vi "Periodic Tasks.vi"() -> ()   [LabVIEW 2014]
doc: "This VI runs in parallel to other tasks. It can contain as many user-defined periodic loops as you need. These can carry out PID or other sorts of timed response."
uses:
  <vilib>/Rock Robotics/WPI/DriverStation/WPI_DriverStationRobotMode2.ctl
  NavX Code/navX-MXP Library/COMMON/TypeDefs/Value TypeDefs/navX Device Registers.ctl
  Global Variables.vi
  Robot Global Data.vi
  <vilib>/addons/control/pid/pid.llb/PID (DBL).vi
  <vilib>/addons/control/pid/NI_PID_pid.lvlib
  <vilib>/Rock Robotics/WPI/DriverStation/WPI_DriverStationStatusErrorCache.ctl
  NavX Code/navX-MXP Library/navX-MXP IMU.lvlib
  <vilib>/Utility/file.llb/Write To Spreadsheet File (DBL).vi
  <vilib>/Utility/file.llb/Read From Spreadsheet File (DBL).vi
panel:
  out "Heading":cluster{"X":dbl, "Y":dbl}[](graph)
  out "Yaw":cluster{"X":dbl, "Y":dbl}[](graph)
  out "Roll":cluster{"X":dbl, "Y":dbl}[](graph)
  out "Pitch":cluster{"X":dbl, "Y":dbl}[](graph)
  in  "Angle":dbl=5.0 format="%#_13g"
  out "Robot Y":dbl
  out "Robot X":dbl
  in  "On Ramp":bool
  in  "Stationary Gryo":dbl
  in  "PID gains":T1={"proportional gain (Kc)"=0.02, "integral time (Ti, min)"=0.0, "derivative time (Td, min)"=0.0} {"derivative time (Td, min)" format="%.3f"; "integral time (Ti, min)" format="%.3f"; "proportional gain (Kc)" format="%.3f"}
  out "Valid?":bool
  out "Offset":dbl
  in  "Left Rumble":sgl
  in  "Right Rumble":sgl
  out "navX Data":u8[](array[numeric])
  in  "PID gains":T1={"proportional gain (Kc)"=1.0, "integral time (Ti, min)"=0.01, "derivative time (Td, min)"=0.0} {"derivative time (Td, min)" format="%.3f"; "integral time (Ti, min)" format="%.3f"; "proportional gain (Kc)" format="%.3f"}
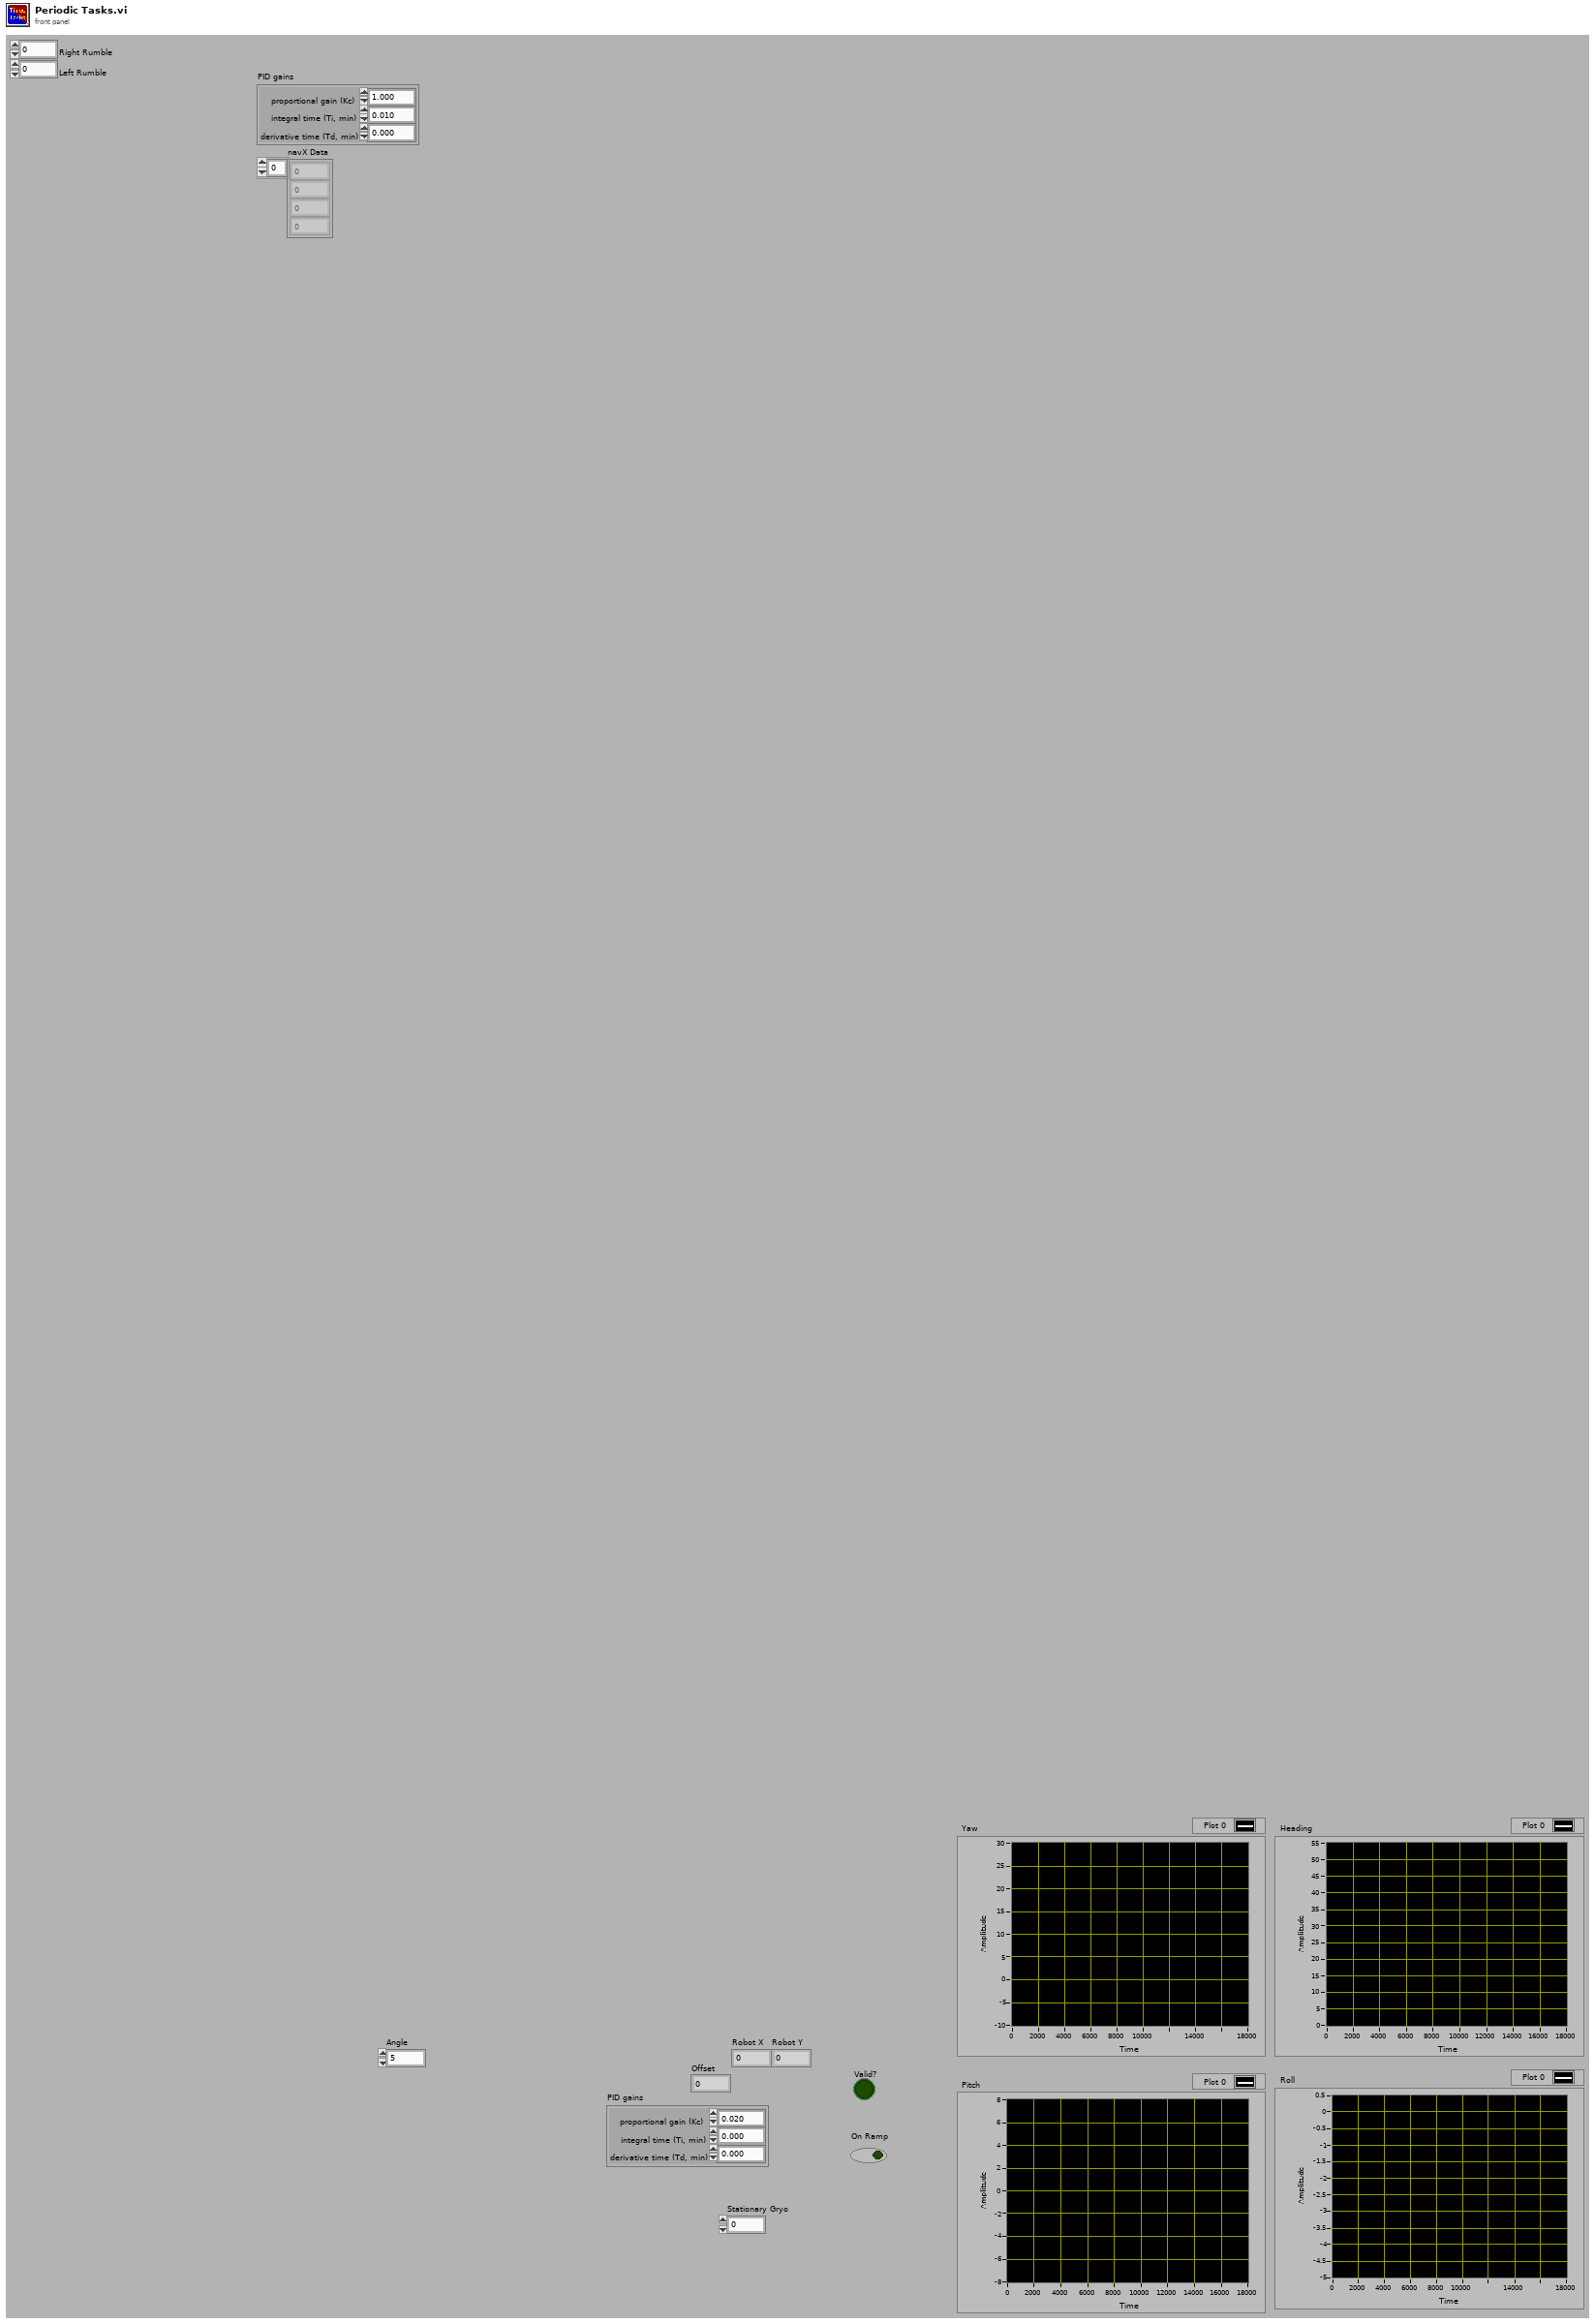
[diagram p1: front panel]
types:
  T1 = cluster{"proportional gain (Kc)":dbl, "integral time (Ti, min)":dbl, "derivative time (Td, min)":dbl}
  T2 = enum16{"Stop", "Three Tote", "Two Tote", "One Tote", "Step", "Top", "Home", "Joystick"}
  T3 = typedef "WPI_JoystickDevRef.ctl" = cluster{"Device":T4}
  T4 = typedef "WPI_JoystickDeviceEnum.ctl" = enum16{"USB 0", "USB 1", "USB 2", "USB 3", "USB 4", "USB 5"}
  T5 = typedef "navX-MXP IMU.lvlib/navX Device Registers.ctl" = u8
  T6 = typedef "navX-MXP IMU.lvlib/navX Device TypeDef.ctl" = cluster{"navX Interface Protocol":T7, "navX Interface Protocol TypeDefs":cluster{"SPIDevRef":T8, "I2CDevRef":T11}, "navX System Information":cluster{"Board Information":T13, "Status":T14, "Offsets":T18}, "navX Common Information":cluster{"Update Rate (4Hz-60Hz)":T19, "refnum name":string, "error":errorcluster}}
  T7 = typedef "navX-MXP IMU.lvlib/navX Interface Protocol.ctl" = enum16{"SPI", "I2C"}
  T8 = typedef "WPI_SPIDevRef.ctl" = cluster{"DevStatus":errorcluster, "Handle":i32, "Controller":T9, "SPI Bus":T10}
  T9 = typedef "FPGA_TypedefDigitalModule.ctl" = enum16{"Controller 1"}
  T10 = typedef "spi_bus.ctl" = enum16{"SPI On-Board, CS0", "SPI On-Board, CS1", "SPI On-Board, CS2", "SPI On-Board, CS3", "SPI MXP", "Invalid"}
  T11 = typedef "WPI_I2CDevRef.ctl" = cluster{"DevStatus":errorcluster, "Controller":T9, "Device Address":u8, "Handle":i32, "I2C Bus":T12}
  T12 = typedef "i2c_bus.ctl" = enum16{"I2C On-Board", "I2C MXP", "Invalid"}
  T13 = typedef "navX-MXP IMU.lvlib/navX Board Information.ctl" = cluster{"WhoAmI (50 | 0x32)":u8, "Board Revision":u8, "Firmware Major Version":u8, "Firmware Minor Version":u8}
  T14 = typedef "navX-MXP IMU.lvlib/navX Status Data.ctl" = cluster{"Update Rate Hz":u8, "Accelerometer Full-Scale Range":u8, "Gyro Full-Scale Range":u16, "NAVX_OP_STATUS":T15, "NAVX_CAL_STATUS":T16, "NAVX_SELFTEST_STATUS":u8, "NAVX_SENSOR_STATUS":T17}
  T15 = typedef "navX-MXP IMU.lvlib/navX NAVX_OP_STATUS.ctl" = u8
  T16 = typedef "navX-MXP IMU.lvlib/navX NAVX_CAL_STATUS.ctl" = u8
  T17 = typedef "navX-MXP IMU.lvlib/navX NAVX_SENSOR_STATUS.ctl" = cluster{"MOVING":bool, "YAW_STABLE":bool, "MAG_DISTURBANCE":bool, "ALTITUDE_VALID":bool, "SEALEVEL_PRESS_SET":bool, "FUSED_HEADING_VALID":bool}
  T18 = typedef "navX-MXP IMU.lvlib/navX Offsets Data.ctl" = cluster{"Yaw":dbl, "Quat W":dbl, "Quat X":dbl, "Quat Y":dbl, "Quat Z":dbl}
  T19 = typedef "navX-MXP IMU.lvlib/navX Update Rate.ctl" = u8
  T20 = typedef "WPI_DriverStationStatusErrorCache.ctl" = enum16{"Get", "Set"}
  T21 = typedef "WPI_MotorControlDeviceRef.ctl" = cluster{"DeviceStatus":errorcluster, "Type":T22, "PWM":cluster{"Controller":T9, "PWM Channel":T23, "DeadBand":T24}, "CAN":cluster{"Device Number":u8, "Control Mode":T25, "Semaphore":T26, "Max Vout":dbl, "TalonSRX Control Mode":T27}, "Invert":bool, "TransformRef":T28, "InvTransformRef":T28}
  T22 = typedef "WPI_MotorControlType.ctl" = enum16{"PWM", "CAN", "CANTalonSRX"}
  T23 = typedef "FPGA_DIOPWMChannel.ctl" = enum8{"PWM 0", "PWM 1", "PWM 2", "PWM 3", "PWM 4", "PWM 5", "PWM 6", "PWM 7", "PWM 8", "PWM 9", "PWM MXP 0", "PWM MXP 1", "PWM MXP 2", "PWM MXP 3", "PWM MXP 4", "PWM MXP 5", "PWM MXP 6", "PWM MXP 7", "PWM MXP 8", "PWM MXP 9", "Invalid"}
  T24 = typedef "WPI_PWMDeadband.ctl" = cluster{"Name":string, "maxPositivePwm":i32, "minPositivePwm":i32, "centerPwm":i32, "maxNegativePwm":i32, "minNegativePwm":i32, "angularRange":u16}
  T25 = typedef "WPI_CANJaguar_ControlMode.ctl" = enum8{"Percent VBus", "Current", "Speed", "Position", "Voltage"}
  T26 = typedef "Semaphore RefNum" = refnum<k1>
  T27 = typedef "WPI_CANTalonSRX_APIControlMode.ctl" = enum8{"Percent VBus", "Speed", "Position", "Slave", "Unchanged / Invalid"}
  T28 = typedef "WPI_PWMTransform_ConPane.ctl" = refnum<vi>
  T29 = typedef "WPI_DriverStationRobotMode2.ctl" = enum16{"Autonomous Disabled", "Autonomous Enabled", "Teleop Disabled", "Teleop Enabled", "Disconnected", "Finish", "Test Disabled", "Test Enabled", "Emergency Stopped"}
  T30 = typedef "navX-MXP IMU.lvlib/navX Vector Data.ctl" = cluster{"X":dbl, "Y":dbl, "Z":dbl}
  T31 = typedef "navX-MXP IMU.lvlib/navX YPRH Data.ctl" = cluster{"Yaw":dbl, "Pitch":dbl, "Roll":dbl, "Heading":dbl}
  T32 = typedef "WPI_CounterDevRef.ctl" = cluster{"DevStatus":errorcluster, "CntIndex":T33}
  T33 = typedef "FPGA_CounterCtrSystemIndex.ctl" = enum8{"Ctr 0", "Ctr 1", "Ctr 2", "Ctr 3", "Ctr 4", "Ctr 5", "Ctr 6", "Ctr 7", "Invalid"}
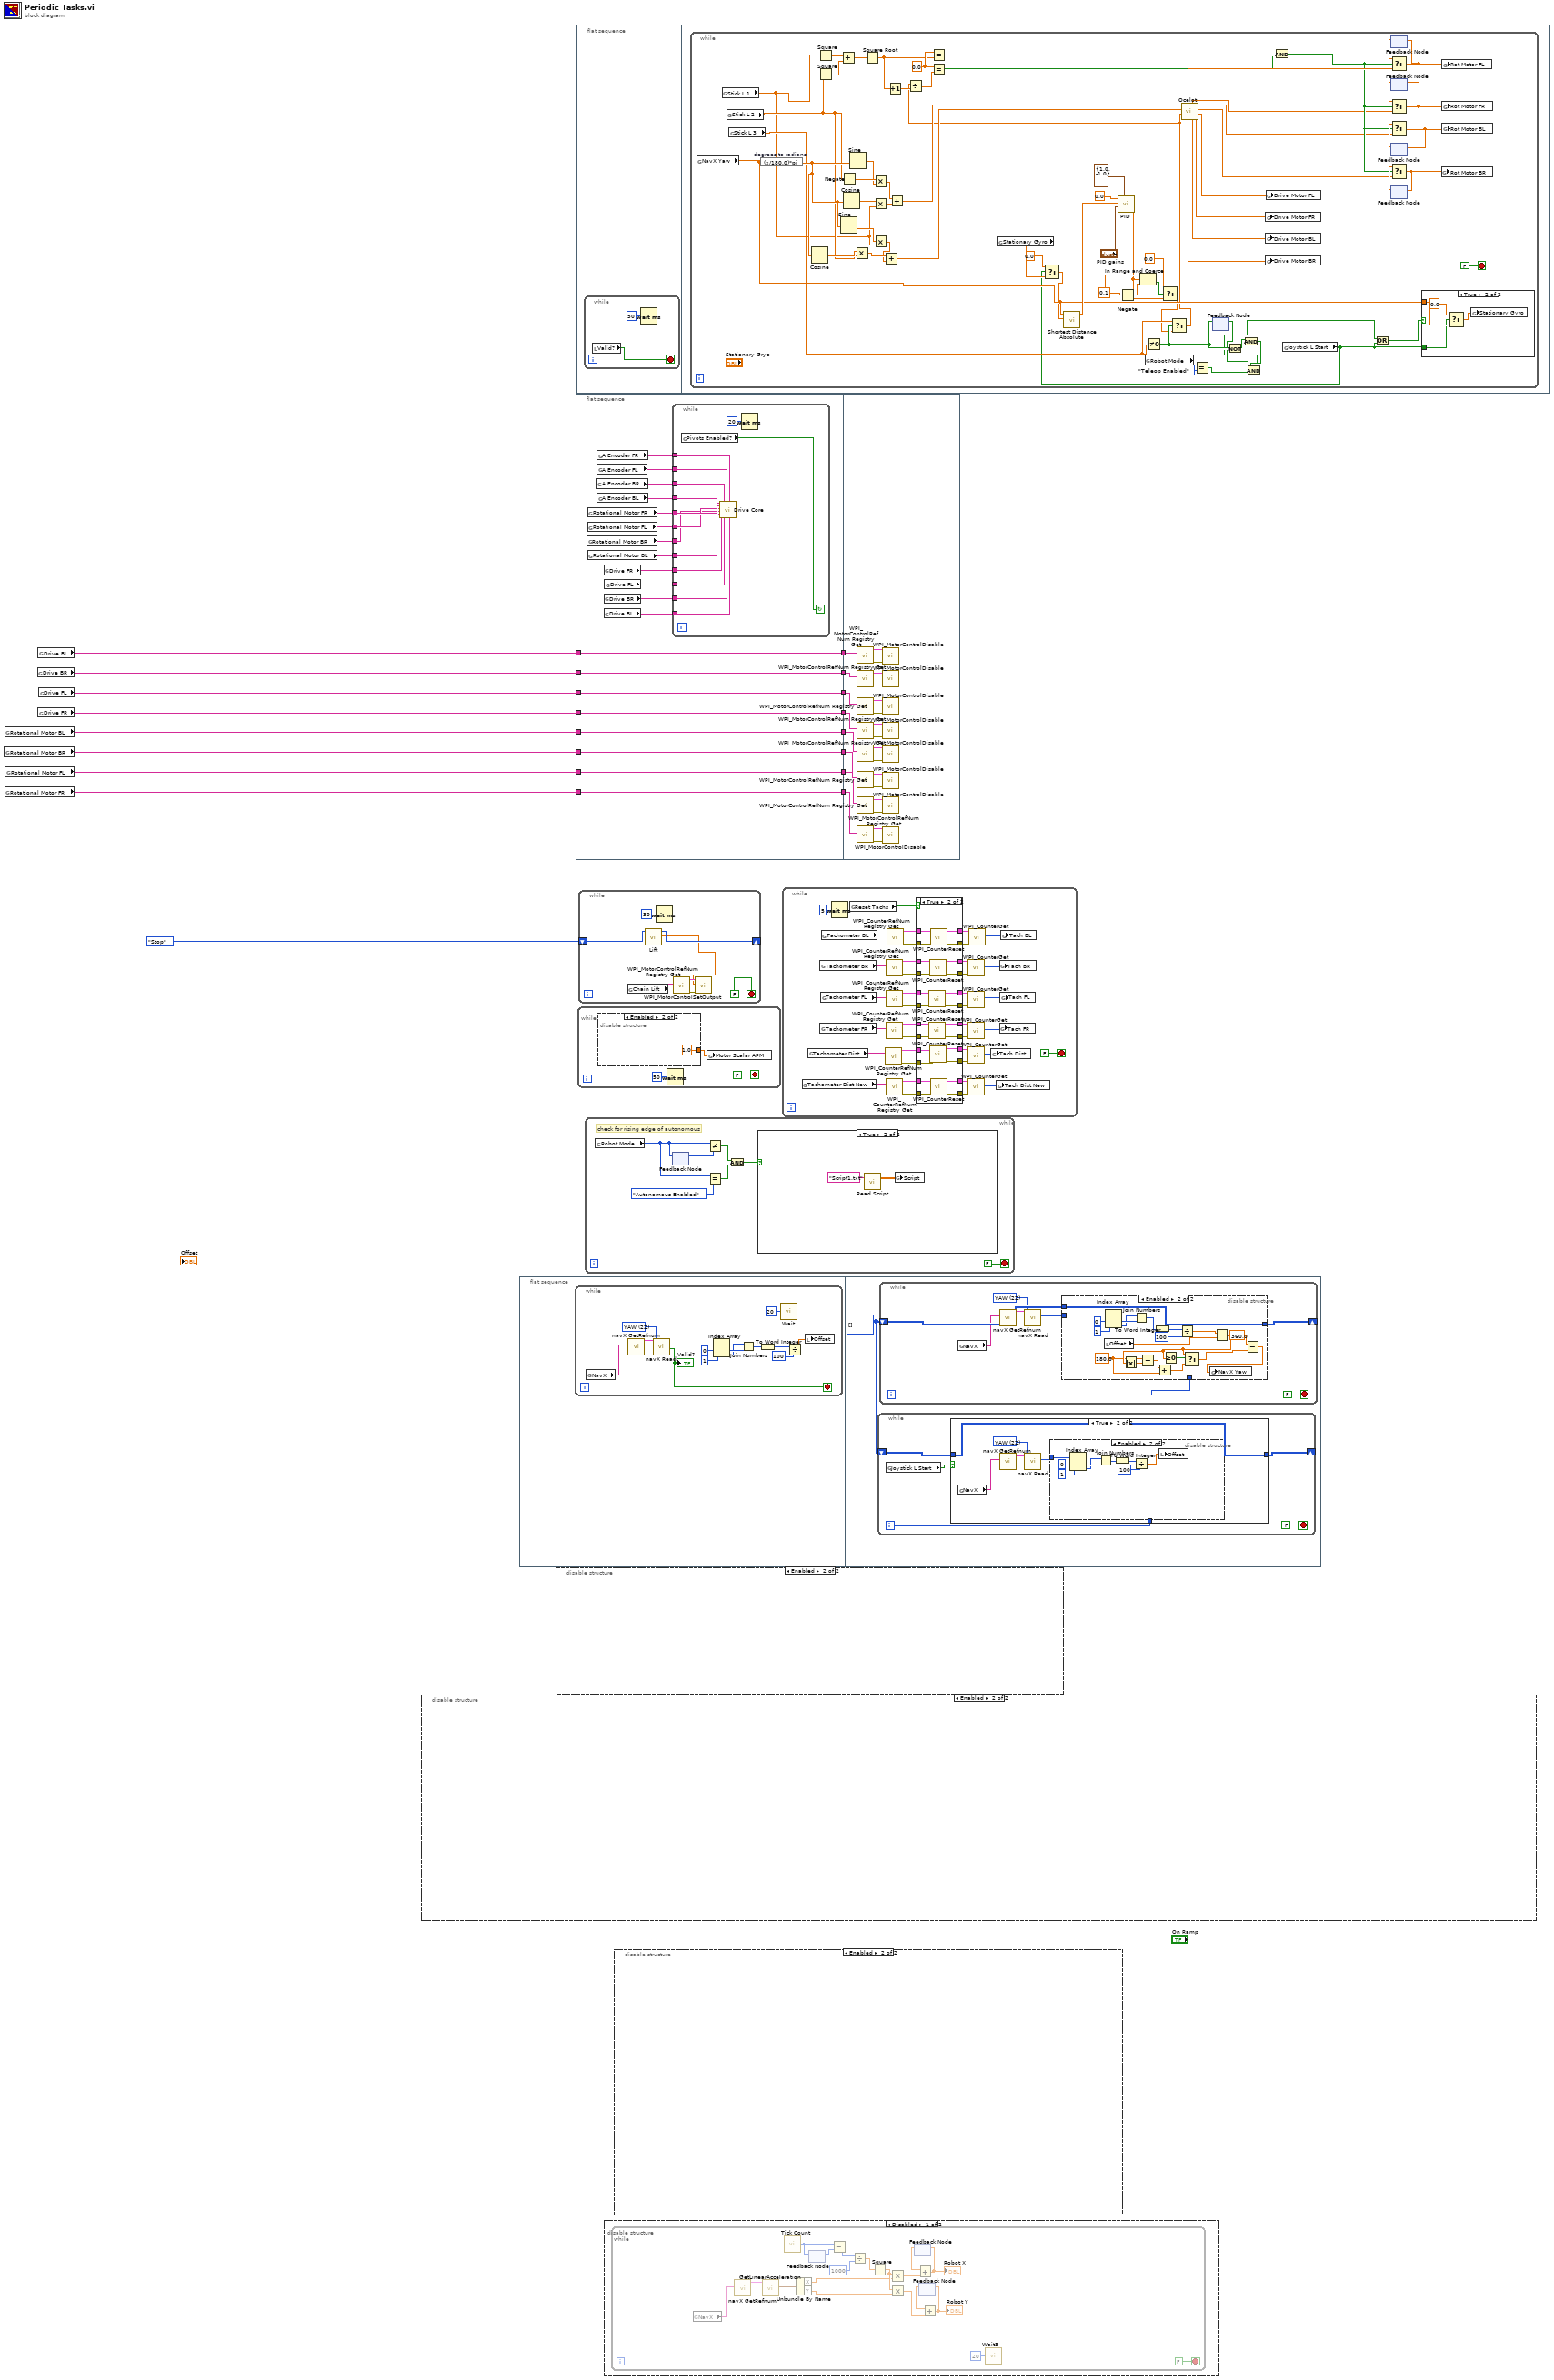
[diagram p0: block diagram]
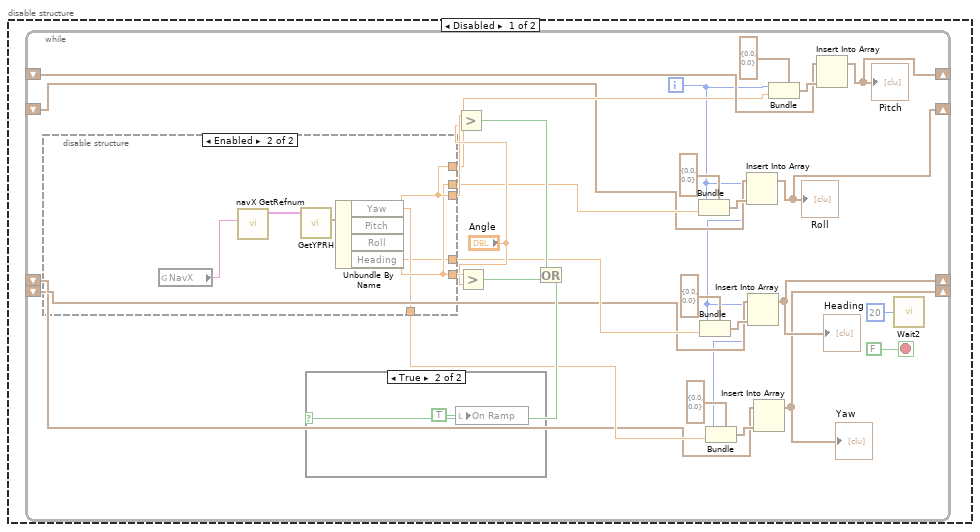
[diagram p4: hidden frame]
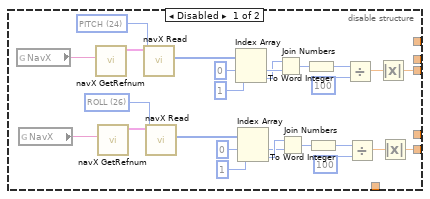
[diagram p5: hidden frame]
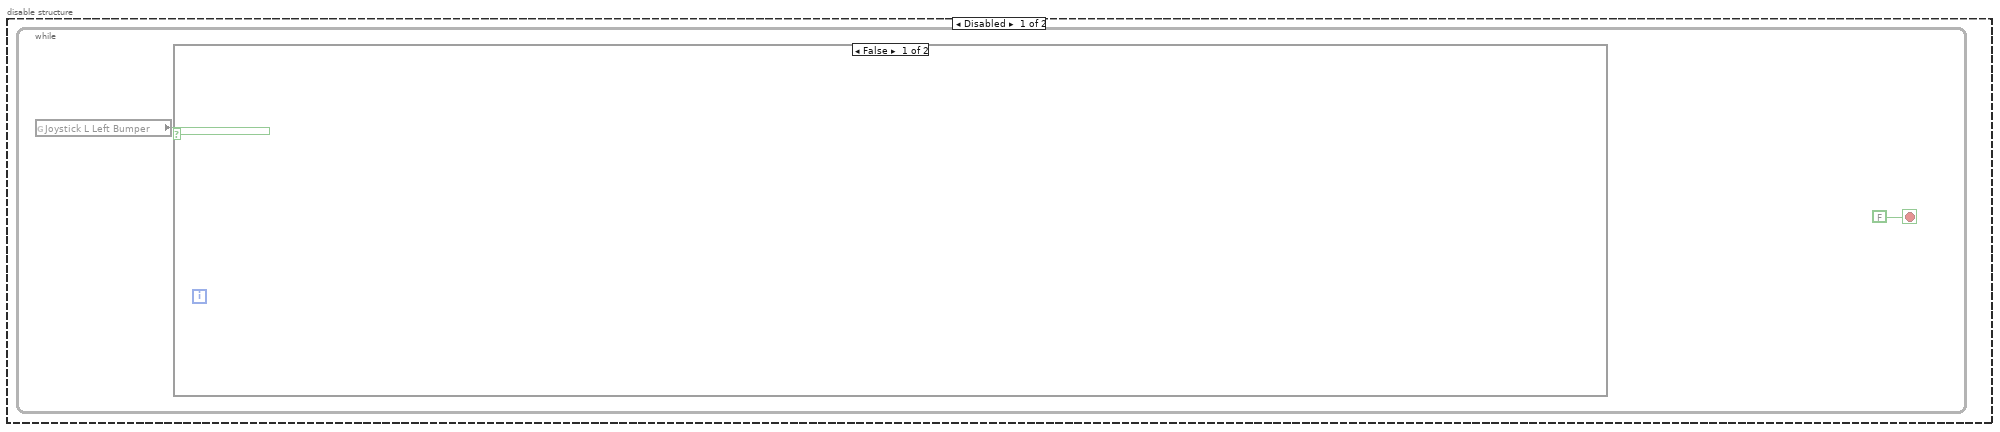
[diagram p7: hidden frame]
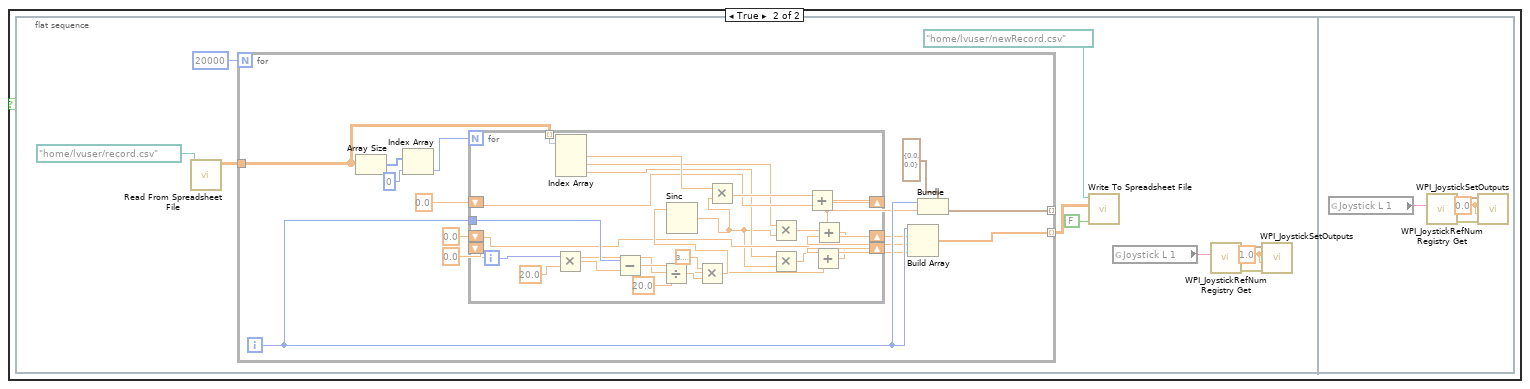
[diagram p8: hidden frame]
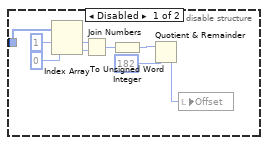
[diagram p10: hidden frame]
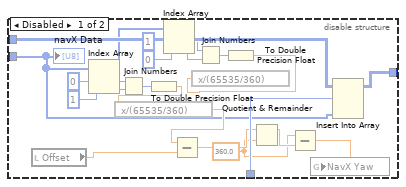
[diagram p11: hidden frame]
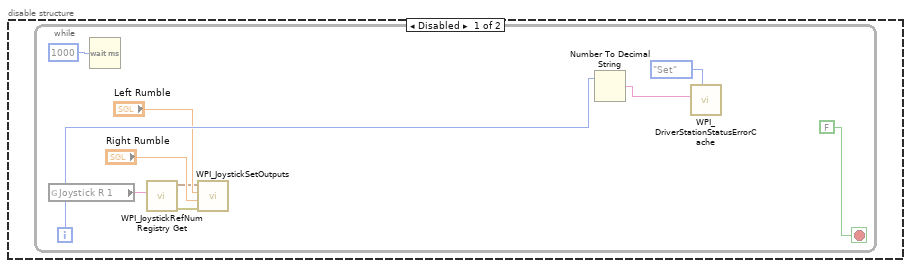
[diagram p12: hidden frame]
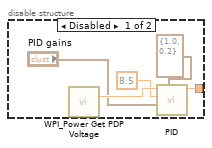
[diagram p15: hidden frame]
diagram:
  n1 = global read "Global Variables.vi" "Rotational Motor BR"() -> (w6:string)
  n2 = global read "Global Variables.vi" "Rotational Motor BL"() -> (w8:string)
  n3 = global read "Global Variables.vi" "Rotational Motor FR"() -> (w2:string)
  n4 = global read "Global Variables.vi" "Rotational Motor FL"() -> (w4:string)
  n5 = global read "Global Variables.vi" "Drive BR"() -> (w14:string)
  n6 = global read "Global Variables.vi" "Drive BL"() -> (w16:string)
  n7 = global read "Global Variables.vi" "Drive FR"() -> (w10:string)
  n8 = global read "Global Variables.vi" "Drive FL"() -> (w12:string)
  n9 = disable-structure shown="Enabled" {
    frame Disabled {
      n10 = while {
        stop <- FALSE stop-if-true
        n11 = global read "Global Variables.vi" "Joystick L Left Bumper"() -> (w18:bool)
        n12 = case shown="False" w18 {
          frame False {
          }
          frame True {
            n13 = flat-sequence {
              frame #0 {
                w23 = sgl 1.0 ("Left Rumble")
                n14 = call-poly <vilib>:"Read From Spreadsheet File.vi"("file path (dialog if empty)"=path "/home/lvuser/record.csv") -> ("all rows"=w28:dbl[][])  [unwired: 6 in, 4 out]
                n15 = for {
                  N: 20000 -> [_]
                  tunnel: [w38] -> _ mode=indexing
                  tunnel: w28 -> [w37]
                  tunnel: [w34] -> w27 mode=indexing
                  i -> [w36]
                  n16 = Array Size(array=w37) -> (size(s)=w43:i32[])
                  n17 = Index Array(array=w43, index=0) -> (element=w42:i32)
                  n18 = for {
                    N: w42 -> [_]
                    shift-right: [w53] -> w35
                    shift-left: 0.0 -> [w55]
                    tunnel: w37 -> [w64] mode=indexing
                    tunnel: w36 -> [w56]
                    shift-right: [w51] -> w33
                    shift-left: 0.0 -> [w48]
                    shift-right: [w52] -> w32
                    shift-left: 0.0 -> [w47]
                    i -> [w62]
                    n19 = Multiply(x=w62, y=20.0) -> (x*y=w59:dbl)
                    n20 = Index Array(array=w64) -> (element #1=w65:dbl, element #2=w46:dbl, element #3=w45:dbl)  [unwired: 3 in]
                    n21 = Subtract(x=w56, y=w59) -> (x-y=w61:dbl)
                    n22 = Divide(x=w61, y=20.0) -> (x/y=w58:dbl)
                    n23 = Multiply(x=3.141592653589793, y=w58) -> (x*y=w54:dbl)
                    n24 = Sinc(1:w54) -> (0:w44:dbl)
                    n25 = Multiply(x=w65, y=w44) -> (x*y=w66:dbl)
                    n26 = Multiply(x=w46, y=w44) -> (x*y=w49:dbl)
                    n27 = Multiply(x=w45, y=w44) -> (x*y=w50:dbl)
                    n28 = Add(x=w66, y=w55) -> (x+y=w53:dbl)
                    n29 = Add(x=w50, y=w47) -> (x+y=w52:dbl)
                    n30 = Add(x=w49, y=w48) -> (x+y=w51:dbl)
                  }
                  n31 = Build Array(w36, w35, w33, w32) -> (w34:dbl[])
                  n32 = Bundle(cluster=cluster{dbl, dbl} {0.0, 0.0}, w36, w35) -> (w38:cluster{dbl, dbl})
                }
                n33 = call-poly <vilib>:"Write To Spreadsheet File.vi"("append to file? (new file:F)"=FALSE, "2D data"=w27, "file path (dialog if empty)"=path "/home/lvuser/newRecord.csv") -> ()  [unwired: 5 in, 1 out]
                n34 = global read "Global Variables.vi" "Joystick L 1"() -> (w21:string)
                n35 = call <vilib>:"WPI_JoystickRefNum Registry Get.vi"("refnum name"=w21) -> ("error out"=w20:errorcluster, "JoystickDevRef"=w22:T3)  [unwired: 9 in]
                n36 = call <vilib>:"WPI_JoystickSetOutputs.vi"("error in (no error)"=w20, "Right Rumble"=w23, "Left Rumble"=w23, "JoystickDevRef"=w22) -> ()  [unwired: 6 in, 2 out]
              }
              frame #1 {
                w67 = sgl 0.0 ("Left Rumble")
                n37 = global read "Global Variables.vi" "Joystick L 1"() -> (w69:string)
                n38 = call <vilib>:"WPI_JoystickRefNum Registry Get.vi"("refnum name"=w69) -> ("error out"=w70:errorcluster, "JoystickDevRef"=w68:T3)  [unwired: 9 in]
                n39 = call <vilib>:"WPI_JoystickSetOutputs.vi"("error in (no error)"=w70, "Right Rumble"=w67, "Left Rumble"=w67, "JoystickDevRef"=w68) -> ()  [unwired: 6 in, 2 out]
              }
            }
          }
        }
      }
    }
    frame Enabled {
    }
  }
  n40 = flat-sequence {
    frame #0 {
      n41 = while {
        stop <- w72 stop-if-true
        w84 = T5 22 items=["WHOAMI"=0, "HW_REV"=1, "FW_VER_MAJOR"=2, "FW_VER_MINOR"=3, "UPDATE_RATE_HZ"=4, "ACCEL_FSR_G"=5, "GYRO_FSR_DPS"=6, "OP_STATUS"=8, "CAL_STATUS"=9, "SELFTEST_STATUS"=10, "SENSOR_STATUS"=16, "TIMESTAMP"=18, "YAW"=22, "PITCH"=24, "ROLL"=26, "HEADING"=28, "FUSED_HEADING"=30, "ALTITUDE_I"=32, "ALTITUDE_D"=34, "LINERA_ACC_X"=36, "LINERA_ACC_Y"=38, "LINERA_ACC_Z"=40, "QUAT_W"=42, "QUAT_X"=44, "QUAT_Y"=46, "QUAT_Z"=48, "MPU_TEMP_C"=50, "GYRO_X"=52, "GYRO_Y"=54, "GYRO_Z"=56, "ACC_X"=58, "ACC_Y"=60, "ACC_Z"=62, "MAG_X"=64, "MAG_Y"=66, "MAG_Z"=68, "PRESSURE_I"=70, "PRESSURE_D"=72, "PRESSURE_TEMP"=74, "YAW_OFFSET"=76, "QUAT_OFFSET_W"=78, "QUAT_OFFSET_X"=80, "QUAT_OFFSET_Y"=82, "QUAT_OFFSET_Z"=84] ("Device Register (WHOAMI)")
        n42 = global read "Global Variables.vi" "NavX"() -> (w83:string)
        n43 = call "navX GetRefnum.vi"("refnum name"=w83) -> ("navX Device TypeDef"=w82:T6)  [unwired: 9 in, 1 out]
        n44 = call "navX Read.vi"("Device Register (WHOAMI)"=w84, "navX Device TypeDef"=w82) -> ("Valid?"=w72:bool, "navX Data"=w81:u8[])  [unwired: 7 in, 1 out]
        "Valid?" <- w72
        n45 = Index Array(array=w81, index #1=0 ("index"), index #2=1 ("index")) -> (element #1=w75:u8, element #2=w74:u8)
        n46 = Join Numbers(hi=w74, lo=w75) -> ((hi.lo)=w78:u16)
        n47 = To Word Integer(number=w78) -> (16bit integer=w77:i16)
        n48 = call "Wait"("Count(mSec)"=u32 20) -> ()  [unwired: 1 out]
        n49 = Divide(x=w77, y=i16 100) -> (x/y=w71:dbl)
        n50 = local write "Offset"(w71) -> ()
      }
    }
    frame #1 {
      w85 = u16[][] []
      n51 = while {
        shift-right: [w88] -> _
        shift-left: w85 -> [w87]
        i -> [w89]
        stop <- FALSE stop-if-true
        n52 = global read "Global Variables.vi" "Joystick L Start"() -> (w86:bool)
        n53 = case shown="True" w86 {
          tunnel: w89 -> [_ _]
          tunnel: [w91 w92] -> w88
          tunnel: w87 -> [w91 w92]
          frame False {
          }
          frame True {
            w94 = T5 22 items=["WHOAMI"=0, "HW_REV"=1, "FW_VER_MAJOR"=2, "FW_VER_MINOR"=3, "UPDATE_RATE_HZ"=4, "ACCEL_FSR_G"=5, "GYRO_FSR_DPS"=6, "OP_STATUS"=8, "CAL_STATUS"=9, "SELFTEST_STATUS"=10, "SENSOR_STATUS"=16, "TIMESTAMP"=18, "YAW"=22, "PITCH"=24, "ROLL"=26, "HEADING"=28, "FUSED_HEADING"=30, "ALTITUDE_I"=32, "ALTITUDE_D"=34, "LINERA_ACC_X"=36, "LINERA_ACC_Y"=38, "LINERA_ACC_Z"=40, "QUAT_W"=42, "QUAT_X"=44, "QUAT_Y"=46, "QUAT_Z"=48, "MPU_TEMP_C"=50, "GYRO_X"=52, "GYRO_Y"=54, "GYRO_Z"=56, "ACC_X"=58, "ACC_Y"=60, "ACC_Z"=62, "MAG_X"=64, "MAG_Y"=66, "MAG_Z"=68, "PRESSURE_I"=70, "PRESSURE_D"=72, "PRESSURE_TEMP"=74, "YAW_OFFSET"=76, "QUAT_OFFSET_W"=78, "QUAT_OFFSET_X"=80, "QUAT_OFFSET_Y"=82, "QUAT_OFFSET_Z"=84] ("Device Register (WHOAMI)")
            n54 = global read "Global Variables.vi" "NavX"() -> (w95:string)
            n55 = call "navX GetRefnum.vi"("refnum name"=w95) -> ("navX Device TypeDef"=w96:T6)  [unwired: 9 in, 1 out]
            n56 = call "navX Read.vi"("Device Register (WHOAMI)"=w94, "navX Device TypeDef"=w96) -> ("navX Data"=w93:u8[])  [unwired: 7 in, 2 out]
            n57 = disable-structure shown="Enabled" {
              disable-tunnel: w93 -> [w100 w109]
              frame Disabled {
                n58 = Index Array(array=w100, index #1=1 ("index"), index #2=0 ("index")) -> (element #1=w99:u8, element #2=w98:u8)
                n59 = Join Numbers(hi=w99, lo=w98) -> ((hi.lo)=w103:u16)
                n60 = To Unsigned Word Integer(number=w103) -> (unsigned 16bit integer=w102:u16)
                n61 = Quotient & Remainder(x=w102, y=u16 182) -> (floor(x/y)=w97:u16)  [unwired: 1 out]
                n62 = local write "Offset"(w97) -> ()
              }
              frame Enabled {
                n63 = Index Array(array=w109, index #1=0 ("index"), index #2=1 ("index")) -> (element #1=w108:u8, element #2=w107:u8)
                n64 = Join Numbers(hi=w107, lo=w108) -> ((hi.lo)=w112:u16)
                n65 = To Word Integer(number=w112) -> (16bit integer=w111:i16)
                n66 = Divide(x=w111, y=i16 100) -> (x/y=w106:dbl)
                n67 = local write "Offset"(w106) -> ()
              }
            }
          }
        }
      }
      n68 = while {
        shift-right: [w120] -> _
        shift-left: w85 -> [w119]
        i -> [w121]
        stop <- FALSE stop-if-true
        w116 = T5 22 items=["WHOAMI"=0, "HW_REV"=1, "FW_VER_MAJOR"=2, "FW_VER_MINOR"=3, "UPDATE_RATE_HZ"=4, "ACCEL_FSR_G"=5, "GYRO_FSR_DPS"=6, "OP_STATUS"=8, "CAL_STATUS"=9, "SELFTEST_STATUS"=10, "SENSOR_STATUS"=16, "TIMESTAMP"=18, "YAW"=22, "PITCH"=24, "ROLL"=26, "HEADING"=28, "FUSED_HEADING"=30, "ALTITUDE_I"=32, "ALTITUDE_D"=34, "LINERA_ACC_X"=36, "LINERA_ACC_Y"=38, "LINERA_ACC_Z"=40, "QUAT_W"=42, "QUAT_X"=44, "QUAT_Y"=46, "QUAT_Z"=48, "MPU_TEMP_C"=50, "GYRO_X"=52, "GYRO_Y"=54, "GYRO_Z"=56, "ACC_X"=58, "ACC_Y"=60, "ACC_Z"=62, "MAG_X"=64, "MAG_Y"=66, "MAG_Z"=68, "PRESSURE_I"=70, "PRESSURE_D"=72, "PRESSURE_TEMP"=74, "YAW_OFFSET"=76, "QUAT_OFFSET_W"=78, "QUAT_OFFSET_X"=80, "QUAT_OFFSET_Y"=82, "QUAT_OFFSET_Z"=84] ("Device Register (WHOAMI)")
        n69 = global read "Global Variables.vi" "NavX"() -> (w117:string)
        n70 = call "navX GetRefnum.vi"("refnum name"=w117) -> ("navX Device TypeDef"=w118:T6)  [unwired: 9 in, 1 out]
        n71 = call "navX Read.vi"("Device Register (WHOAMI)"=w116, "navX Device TypeDef"=w118) -> ("navX Data"=w115:u8[])  [unwired: 7 in, 2 out]
        n72 = disable-structure shown="Enabled" {
          disable-tunnel: w121 -> [w139 _]
          disable-tunnel: [w138 w163] -> w120
          disable-tunnel: w119 -> [w137 w163]
          disable-tunnel: w115 -> [w127 w164]
          frame Disabled {
            w133 = 360.0 ("y")
            n73 = local read "Offset"() -> (w136:dbl)
            n74 = Index Array(array=w127, index #1=0 ("index"), index #2=1 ("index")) -> (element #1=w144:u8, element #2=w143:u8)
            n75 = Join Numbers(hi=w144, lo=w143) -> ((hi.lo)=w140:u16)
            n76 = To Double Precision Float(number=w140) -> (double precision float=w131:dbl)
            n77 = expression code="x/(65535/360)"(w131) -> (w130:dbl)
            n78 = Index Array(array=w127, index #1=1 ("index"), index #2=0 ("index")) -> (element #1=w125:u8, element #2=w124:u8)
            n79 = Subtract(x=w130, y=w136) -> (x-y=w135:dbl)
            n80 = Join Numbers(hi=w125, lo=w124) -> ((hi.lo)=w126:u16)
            n81 = To Double Precision Float(number=w126) -> (double precision float=w123:dbl)
            n82 = expression code="x/(65535/360)"(w123) -> ()  [unwired: 1 out]
            n83 = Quotient & Remainder(x=w135, y=w133) -> (x-y*floor(x/y)=w134:dbl)  [unwired: 1 out]
            n84 = Subtract(x=w133, y=w134) -> (x-y=w132:dbl)
            n85 = global write "Global Variables.vi" "NavX Yaw"(w132) -> ()
            n86 = Insert Into Array(array=w137, index (row)=w139, new element=w127) -> (w138:u16[][])  [unwired: 1 in]
            "navX Data" <- w127
          }
          frame Enabled {
            w148 = 180.0 ("x")
            n87 = local read "Offset"() -> (w156:dbl)
            n88 = Index Array(array=w164, index #1=0 ("index"), index #2=1 ("index")) -> (element #1=w160:u8, element #2=w159:u8)
            n89 = Join Numbers(hi=w159, lo=w160) -> ((hi.lo)=w158:u16)
            n90 = To Word Integer(number=w158) -> (16bit integer=w155:i16)
            n91 = Divide(x=w155, y=i16 100) -> (x/y=w157:dbl)
            n92 = Subtract(x=w157, y=w156) -> (x-y=w152:dbl)
            n93 = Absolute Value(x=w152) -> (abs(x)=w151:dbl)
            n94 = Subtract(x=w148, y=w151) -> (x-y=w149:dbl)
            n95 = Add(x=w149, y=w148) -> (x+y=w150:dbl)
            n96 = Greater Or Equal To 0?(x=w152) -> (x >= 0?=w153:bool)
            n97 = Select(t=w152, s=w153, f=w150) -> (s? t:f=w146:dbl)
            n98 = Subtract(x=360.0, y=w146) -> (x-y=w145:dbl)
            n99 = global write "Global Variables.vi" "NavX Yaw"(w145) -> ()
          }
        }
      }
    }
  }
  n100 = disable-structure shown="Enabled" {
    frame Disabled {
      n101 = while {
        i -> [w171]
        stop <- FALSE stop-if-true
        n102 = global read "Global Variables.vi" "Joystick R 1"() -> (w166:string)
        n103 = Wait (ms)(milliseconds to wait=u32 1000) -> ()  [unwired: 1 out]
        n104 = call <vilib>:"WPI_JoystickRefNum Registry Get.vi"("refnum name"=w166) -> ("error out"=w165:errorcluster, "JoystickDevRef"=w167:T3)  [unwired: 9 in]
        n105 = call <vilib>:"WPI_JoystickSetOutputs.vi"("error in (no error)"=w165, "Right Rumble"="Right Rumble", "Left Rumble"="Left Rumble", "JoystickDevRef"=w167) -> ()  [unwired: 6 in, 2 out]
        n106 = Number To Decimal String(number=w171) -> (decimal integer string=w172:string)  [unwired: 1 in]
        n107 = call <vilib>:"WPI_DriverStationStatusErrorCache.vi"("StatusErrorCacheOp"=WPI_DriverStationStatusErrorCache."Set", "Error String"=w172) -> ()  [unwired: 1 in, 9 out]
      }
    }
    frame Enabled {
    }
  }
  n108 = flat-sequence {
    tunnel: [w182] -> w17
    tunnel: w16 -> [w182]
    tunnel: [w181] -> w15
    tunnel: w14 -> [w181]
    tunnel: [w180] -> w13
    tunnel: w12 -> [w180]
    tunnel: [w179] -> w11
    tunnel: w10 -> [w179]
    tunnel: [w178] -> w9
    tunnel: w8 -> [w178]
    tunnel: [w177] -> w7
    tunnel: w6 -> [w177]
    tunnel: [w176] -> w5
    tunnel: w4 -> [w176]
    tunnel: [w175] -> w3
    tunnel: w2 -> [w175]
    tunnel: w17 -> [w216]
    tunnel: w15 -> [w215]
    tunnel: w13 -> [w214]
    tunnel: w11 -> [w213]
    tunnel: w9 -> [w212]
    tunnel: w7 -> [w211]
    tunnel: w5 -> [w210]
    tunnel: w3 -> [w209]
    frame #0 {
      n109 = global read "Global Variables.vi" "Rotational Motor BR"() -> (w188:string)
      n110 = global read "Global Variables.vi" "Rotational Motor FR"() -> (w190:string)
      n111 = global read "Global Variables.vi" "Rotational Motor FL"() -> (w189:string)
      n112 = global read "Global Variables.vi" "Rotational Motor BL"() -> (w187:string)
      n113 = global read "Global Variables.vi" "A Encoder BR"() -> (w192:string)
      n114 = global read "Global Variables.vi" "A Encoder FR"() -> (w194:string)
      n115 = global read "Global Variables.vi" "A Encoder FL"() -> (w193:string)
      n116 = global read "Global Variables.vi" "A Encoder BL"() -> (w191:string)
      n117 = global read "Global Variables.vi" "Drive FR"() -> (w186:string)
      n118 = global read "Global Variables.vi" "Drive BR"() -> (w184:string)
      n119 = global read "Global Variables.vi" "Drive BL"() -> (w183:string)
      n120 = global read "Global Variables.vi" "Drive FL"() -> (w185:string)
      n121 = while {
        tunnel: w194 -> [w207]
        tunnel: w193 -> [w206]
        tunnel: w192 -> [w205]
        tunnel: w191 -> [w204]
        tunnel: w190 -> [w203]
        tunnel: w189 -> [w202]
        tunnel: w188 -> [w201]
        tunnel: w187 -> [w200]
        tunnel: w186 -> [w199]
        tunnel: w185 -> [w198]
        tunnel: w184 -> [w197]
        tunnel: w183 -> [w196]
        stop <- w208 continue-if-true
        n122 = global read "Global Variables.vi" "Pivots Enabled?"() -> (w208:bool)
        n123 = call "Drive Core.vi"("A Encoder BL"=w204, "Rotational Motor FR"=w203, "Rotational Motor FL"=w202, "Rotational Motor BR"=w201, "Rotational Motor BL"=w200, "Drive Motor FR"=w199, "A Encoder BR"=w205, "Drive Motor FL"=w198, "A Encoder FL"=w206, "Drive Motor BR"=w197, "A Encoder FR"=w207, "Drive Motor BL"=w196) -> ()  [unwired: 8 in]
        n124 = Wait (ms)(milliseconds to wait=u32 20) -> ()  [unwired: 1 out]
      }
    }
    frame #1 {
      n125 = call <vilib>:"WPI_MotorControlRefNum Registry Get.vi"("refnum name"=w216) -> ("error out"=w232:errorcluster, "MotorControlDevRef"=w231:T21)  [unwired: 9 in]
      n126 = call <vilib>:"WPI_MotorControlRefNum Registry Get.vi"("refnum name"=w215) -> ("error out"=w230:errorcluster, "MotorControlDevRef"=w229:T21)  [unwired: 9 in]
      n127 = call <vilib>:"WPI_MotorControlRefNum Registry Get.vi"("refnum name"=w214) -> ("error out"=w228:errorcluster, "MotorControlDevRef"=w227:T21)  [unwired: 9 in]
      n128 = call <vilib>:"WPI_MotorControlRefNum Registry Get.vi"("refnum name"=w213) -> ("error out"=w226:errorcluster, "MotorControlDevRef"=w225:T21)  [unwired: 9 in]
      n129 = call <vilib>:"WPI_MotorControlRefNum Registry Get.vi"("refnum name"=w212) -> ("error out"=w224:errorcluster, "MotorControlDevRef"=w223:T21)  [unwired: 9 in]
      n130 = call <vilib>:"WPI_MotorControlRefNum Registry Get.vi"("refnum name"=w211) -> ("error out"=w222:errorcluster, "MotorControlDevRef"=w221:T21)  [unwired: 9 in]
      n131 = call <vilib>:"WPI_MotorControlRefNum Registry Get.vi"("refnum name"=w210) -> ("error out"=w220:errorcluster, "MotorControlDevRef"=w219:T21)  [unwired: 9 in]
      n132 = call <vilib>:"WPI_MotorControlRefNum Registry Get.vi"("refnum name"=w209) -> ("error out"=w218:errorcluster, "MotorControlDevRef"=w217:T21)  [unwired: 9 in]
      n133 = call <vilib>:"WPI_MotorControlDisable.vi"("error in (no error)"=w232, "MotorControlDevRef"=w231) -> ()  [unwired: 8 in, 2 out]
      n134 = call <vilib>:"WPI_MotorControlDisable.vi"("error in (no error)"=w230, "MotorControlDevRef"=w229) -> ()  [unwired: 8 in, 2 out]
      n135 = call <vilib>:"WPI_MotorControlDisable.vi"("error in (no error)"=w228, "MotorControlDevRef"=w227) -> ()  [unwired: 8 in, 2 out]
      n136 = call <vilib>:"WPI_MotorControlDisable.vi"("error in (no error)"=w226, "MotorControlDevRef"=w225) -> ()  [unwired: 8 in, 2 out]
      n137 = call <vilib>:"WPI_MotorControlDisable.vi"("error in (no error)"=w224, "MotorControlDevRef"=w223) -> ()  [unwired: 8 in, 2 out]
      n138 = call <vilib>:"WPI_MotorControlDisable.vi"("error in (no error)"=w222, "MotorControlDevRef"=w221) -> ()  [unwired: 8 in, 2 out]
      n139 = call <vilib>:"WPI_MotorControlDisable.vi"("error in (no error)"=w220, "MotorControlDevRef"=w219) -> ()  [unwired: 8 in, 2 out]
      n140 = call <vilib>:"WPI_MotorControlDisable.vi"("error in (no error)"=w218, "MotorControlDevRef"=w217) -> ()  [unwired: 8 in, 2 out]
    }
  }
  n141 = flat-sequence {
    frame #0 {
      n142 = while {
        stop <- w234 stop-if-true
        n143 = local read "Valid?"() -> (w234:bool)
        n144 = Wait (ms)(milliseconds to wait=u32 50) -> ()  [unwired: 1 out]
      }
    }
    frame #1 {
      n145 = while {
        stop <- FALSE stop-if-true
        w246 = 0.1 ("Value to Deadband (default of 0.1)")
        w298 = 0.0 ("x")
        n146 = global read "Global Variables.vi" "NavX Yaw"() -> (w253:dbl)
        n147 = global read "Global Variables.vi" "Stick L 1"() -> (w235:dbl)
        n148 = global read "Global Variables.vi" "Stick L 2"() -> (w259:dbl)
        n149 = global read "Global Variables.vi" "Stick L 3"() -> (w258:dbl)
        n150 = expression code="(x/180.0)*pi" "degrees to radians"(w253) -> (w267:dbl)
        n151 = Cosine(x=w267) -> (cos(x)=w266:dbl)
        n152 = Square(x=w235) -> (x^2=w300:dbl)
        n153 = Square(x=w259) -> (x^2=w301:dbl)
        n154 = Add(x=w300, y=w301) -> (x+y=w299:dbl)
        n155 = Sine(x=w267) -> (sin(x)=w274:dbl)
        n156 = Negate(x=w259) -> (-x=w273:dbl)
        n157 = Cosine(x=w267) -> (cos(x)=w271:dbl)
        n158 = Sine(x=w267) -> (sin(x)=w268:dbl)
        n159 = Multiply(x=w266, y=w259) -> (x*y=w265:dbl)
        n160 = Square Root(x=w299) -> (sqrt(x)=w297:dbl)
        n161 = Multiply(x=w273, y=w268) -> (x*y=w272:dbl)
        n162 = Multiply(x=w271, y=w235) -> (x*y=w270:dbl)
        n163 = Multiply(x=w274, y=w235) -> (x*y=w264:dbl)
        n164 = Add(x=w265, y=w264) -> (x+y=w263:dbl)
        n165 = Increment(x=w297) -> (x+1=w296:dbl)
        n166 = Add(x=w272, y=w270) -> (x+y=w269:dbl)
        n167 = Equal?(x=w298, y=w297) -> (x = y?=w289:bool)
        n168 = global read "Global Variables.vi" "Stationary Gyro"() -> (w237:dbl)
        n169 = Negate(x=w246) -> (-x=w247:dbl)
        n170 = global read "Robot Global Data.vi" "Robot Mode"() -> (w251:T29)
        n171 = Not Equal To 0?(x=w258) -> (x != 0?=w255:bool)
        n172 = Equal?(x=w251, y=WPI_DriverStationRobotMode2."Teleop Enabled") -> (x = y?=w249:bool)
        n173 = feedback #1() -> (w254:bool)  [unwired: 1 in]
        n174 = feedback-in #1(w255) -> ()
        n175 = Not(x=w255) -> (.not. x?=w256:bool)
        n176 = And(x=w256, y=w254) -> (x .and. y?=w248:bool)
        n177 = And(x=w248, y=w249) -> (x .and. y?=w241:bool)
        n178 = global read "Global Variables.vi" "Joystick L Start"() -> (w236:bool)
        n179 = Select(t=0.0, s=w236, f=w237) -> (s? t:f=w238:dbl)
        n180 = call "Shortest Distance Absolute.vi"("Target"=w238, "Current"=w253) -> ("Angle to Rotate"=w257:dbl)  [unwired: 9 in]
        n181 = call-poly <vilib>:"PID.vi"("output range"=cluster{"output high":dbl, "output low":dbl} {"output high"=1.0, "output low"=-1.0}, "PID gains"="PID gains", "process variable"=w257, "setpoint"=0.0) -> ("output"=w243:dbl)  [unwired: 6 in, 1 out]
        n182 = In Range and Coerce(upper limit=w246, x=w243, lower limit=w247) -> (In Range?=w245:bool)  [unwired: 1 out]
        n183 = Select(t=0.0, s=w245, f=w243) -> (s? t:f=w242:dbl)
        n184 = Select(t=w258, s=w255, f=w242) -> (s? t:f=w252:dbl)
        n185 = Divide(x=w252, y=w296) -> (x/y=w295:dbl)
        n186 = Equal?(x=w298, y=w295) -> (x = y?=w288:bool)
        n187 = call "Ocelot.vi"("RCW (X2)"=w252, "FWD (Y)"=w263, "STR (X)"=w269) -> ("FRD"=w278:dbl, "FLD"=w279:dbl, "BRS"=w280:dbl, "BLS"=w281:dbl, "BLD"=w277:dbl, "FRS"=w282:dbl, "BRD"=w276:dbl, "FLS"=w290:dbl)  [unwired: 1 in]
        n188 = global write "Global Variables.vi" "Drive Motor FR"(w278) -> ()
        n189 = global write "Global Variables.vi" "Drive Motor BL"(w277) -> ()
        n190 = global write "Global Variables.vi" "Drive Motor BR"(w276) -> ()
        n191 = global write "Global Variables.vi" "Drive Motor FL"(w279) -> ()
        n192 = And(x=w289, y=w288) -> (x .and. y?=w287:bool)
        n193 = Or(x=w241, y=w236) -> (x .or. y?=w240:bool)
        n194 = feedback #2() -> (w294:dbl)  [unwired: 1 in]
        n195 = Select(t=w294, s=w287, f=w290) -> (s? t:f=w286:dbl)
        n196 = feedback-in #2(w286) -> ()
        n197 = feedback #3() -> (w293:dbl)  [unwired: 1 in]
        n198 = Select(t=w293, s=w287, f=w282) -> (s? t:f=w285:dbl)
        n199 = feedback-in #3(w285) -> ()
        n200 = feedback #4() -> (w292:dbl)  [unwired: 1 in]
        n201 = Select(t=w292, s=w287, f=w281) -> (s? t:f=w284:dbl)
        n202 = feedback-in #4(w284) -> ()
        n203 = feedback #5() -> (w291:dbl)  [unwired: 1 in]
        n204 = Select(t=w291, s=w287, f=w280) -> (s? t:f=w283:dbl)
        n205 = feedback-in #5(w283) -> ()
        n206 = case shown="True" w240 {
          tunnel: w253 -> [_ w305]
          tunnel: w236 -> [_ w304]
          frame False {
          }
          frame True {
            n207 = Select(t=0.0, s=w304, f=w305) -> (s? t:f=w302:dbl)
            n208 = global write "Global Variables.vi" "Stationary Gyro"(w302) -> ()
          }
        }
        n209 = global write "Global Variables.vi" "Rot Motor BR"(w283) -> ()
        n210 = global write "Global Variables.vi" "Rot Motor FL"(w286) -> ()
        n211 = global write "Global Variables.vi" "Rot Motor FR"(w285) -> ()
        n212 = global write "Global Variables.vi" "Rot Motor BL"(w284) -> ()
      }
    }
  }
  n213 = while {
    stop <- FALSE stop-if-true
    n214 = disable-structure shown="Enabled" {
      disable-tunnel: [w309 1.0 ("Motor Scalar APM")] -> w306
      frame Disabled {
        n215 = call <vilib>:"WPI_Power Get PDP Voltage.vi"() -> ("voltage (V)"=w312:dbl)  [unwired: 14 in, 1 out]
        n216 = call-poly <vilib>:"PID.vi"("output range"=cluster{"output high":dbl, "output low":dbl} {"output high"=1.0, "output low"=0.2}, "PID gains"="PID gains", "process variable"=8.5 ("setpoint"), "setpoint"=w312) -> ("output"=w309:dbl)  [unwired: 6 in, 1 out]
      }
      frame Enabled {
      }
    }
    n217 = Wait (ms)(milliseconds to wait=u32 50) -> ()  [unwired: 1 out]
    n218 = global write "Global Variables.vi" "Motor Scalar APM"(w306) -> ()
  }
  n219 = while {
    shift-right: [w320] -> _
    shift-left: T2."Stop" ("State Out") -> [w321]
    stop <- FALSE stop-if-true
    n220 = global read "Global Variables.vi" "Chain Lift"() -> (w315:string)
    n221 = call "Lift.vi"("State"=w321) -> ("Lift Motor(Global...)"=w316:dbl, "State Out"=w320:T2)  [unwired: 9 in]
    n222 = Wait (ms)(milliseconds to wait=u32 30) -> ()  [unwired: 1 out]
    n223 = call <vilib>:"WPI_MotorControlRefNum Registry Get.vi"("refnum name"=w315) -> ("error out"=w319:errorcluster, "MotorControlDevRef"=w318:T21)  [unwired: 9 in]
    n224 = call <vilib>:"WPI_MotorControlSetOutput.vi"("error in (no error)"=w319, "Output"=w316, "MotorControlDevRef"=w318) -> ()  [unwired: 6 in, 3 out]
  }
  n225 = while {
    stop <- FALSE stop-if-true
    # "check for rising edge of autonomous"
    n226 = global read "Robot Global Data.vi" "Robot Mode"() -> (w327:T29)
    n227 = feedback #6() -> (w329:T29)  [unwired: 1 in]
    n228 = feedback-in #6(w327) -> ()
    n229 = Not Equal?(x=w327, y=w329) -> (x != y?=w325:bool)
    n230 = Equal?(x=w327, y=WPI_DriverStationRobotMode2."Autonomous Enabled" ("Robot Mode")) -> (x = y?=w326:bool)
    n231 = And(x=w325, y=w326) -> (x .and. y?=w323:bool)
    n232 = case shown="True" w323 {
      frame False {
      }
      frame True {
        n233 = call "Read Script.vi"("script name"="Script1.txt") -> ("output array"=w330:dbl[][])  [unwired: 1 in, 1 out]
        n234 = global write "Global Variables.vi" "Script"(w330) -> ()
      }
    }
  }
  n235 = disable-structure shown="Disabled" {
    frame Disabled {
      n236 = while {
        stop <- FALSE stop-if-true
        n237 = global read "Global Variables.vi" "NavX"() -> (w349:string)
        n238 = call "navX GetRefnum.vi"("refnum name"=w349) -> ("navX Device TypeDef"=w348:T6)  [unwired: 9 in, 1 out]
        n239 = call "GetLinearAcceleration.vi"("navX Device TypeDef"=w348) -> ("Linear Acceleration"=w347:T30)  [unwired: 8 in, 2 out]
        n240 = call "Tick Count"() -> ("Tick Count(mSec)"=w343:u32)
        n241 = Unbundle By Name(w347) -> ("X"=w340:dbl, "Y"=w339:dbl)
        n242 = feedback-in #7(w343) -> ()
        n243 = feedback #7() -> (w342:u32)  [unwired: 1 in]
        n244 = Subtract(x=w343, y=w342) -> (x-y=w344:u32)
        n245 = Divide(x=w344, y=u32 1000) -> (x/y=w346:dbl)
        n246 = Square(x=w346) -> (x^2=w341:dbl)
        n247 = Multiply(x=w341, y=w340) -> (x*y=w338:dbl)
        n248 = Multiply(x=w341, y=w339) -> (x*y=w334:dbl)
        n249 = feedback #8() -> (w336:dbl)  [unwired: 1 in]
        n250 = Add(x=w336, y=w338) -> (x+y=w337:dbl)
        "Robot X" <- w337
        n251 = feedback-in #8(w337) -> ()
        n252 = feedback #9() -> (w335:dbl)  [unwired: 1 in]
        n253 = Add(x=w335, y=w334) -> (x+y=w333:dbl)
        "Robot Y" <- w333
        n254 = feedback-in #9(w333) -> ()
        n255 = call "Wait3"("Count(mSec)"=u32 20) -> ()  [unwired: 1 out]
      }
    }
    frame Enabled {
    }
  }
  n256 = disable-structure shown="Enabled" {
    frame Disabled {
      n257 = while {
        shift-right: [w369] -> _
        shift-left: _ -> [w368]
        shift-right: [w363] -> _
        shift-left: _ -> [w362]
        shift-right: [w352] -> _
        shift-left: _ -> [w355]
        shift-right: [w351] -> _
        shift-left: _ -> [w354]
        i -> [w353]
        stop <- FALSE stop-if-true
        n258 = disable-structure shown="Enabled" {
          disable-tunnel: [w394 w409] -> w378
          disable-tunnel: [w391 w408] -> w374
          disable-tunnel: [_ w409] -> w367
          disable-tunnel: [_ w408] -> w364
          disable-tunnel: [_ w407] -> w357
          disable-tunnel: [_ w406] -> w356
          frame Disabled {
            w382 = T5 26 items=["WHOAMI"=0, "HW_REV"=1, "FW_VER_MAJOR"=2, "FW_VER_MINOR"=3, "UPDATE_RATE_HZ"=4, "ACCEL_FSR_G"=5, "GYRO_FSR_DPS"=6, "OP_STATUS"=8, "CAL_STATUS"=9, "SELFTEST_STATUS"=10, "SENSOR_STATUS"=16, "TIMESTAMP"=18, "YAW"=22, "PITCH"=24, "ROLL"=26, "HEADING"=28, "FUSED_HEADING"=30, "ALTITUDE_I"=32, "ALTITUDE_D"=34, "LINERA_ACC_X"=36, "LINERA_ACC_Y"=38, "LINERA_ACC_Z"=40, "QUAT_W"=42, "QUAT_X"=44, "QUAT_Y"=46, "QUAT_Z"=48, "MPU_TEMP_C"=50, "GYRO_X"=52, "GYRO_Y"=54, "GYRO_Z"=56, "ACC_X"=58, "ACC_Y"=60, "ACC_Z"=62, "MAG_X"=64, "MAG_Y"=66, "MAG_Z"=68, "PRESSURE_I"=70, "PRESSURE_D"=72, "PRESSURE_TEMP"=74, "YAW_OFFSET"=76, "QUAT_OFFSET_W"=78, "QUAT_OFFSET_X"=80, "QUAT_OFFSET_Y"=82, "QUAT_OFFSET_Z"=84] ("Device Register (WHOAMI)")
            w403 = T5 24 items=["WHOAMI"=0, "HW_REV"=1, "FW_VER_MAJOR"=2, "FW_VER_MINOR"=3, "UPDATE_RATE_HZ"=4, "ACCEL_FSR_G"=5, "GYRO_FSR_DPS"=6, "OP_STATUS"=8, "CAL_STATUS"=9, "SELFTEST_STATUS"=10, "SENSOR_STATUS"=16, "TIMESTAMP"=18, "YAW"=22, "PITCH"=24, "ROLL"=26, "HEADING"=28, "FUSED_HEADING"=30, "ALTITUDE_I"=32, "ALTITUDE_D"=34, "LINERA_ACC_X"=36, "LINERA_ACC_Y"=38, "LINERA_ACC_Z"=40, "QUAT_W"=42, "QUAT_X"=44, "QUAT_Y"=46, "QUAT_Z"=48, "MPU_TEMP_C"=50, "GYRO_X"=52, "GYRO_Y"=54, "GYRO_Z"=56, "ACC_X"=58, "ACC_Y"=60, "ACC_Z"=62, "MAG_X"=64, "MAG_Y"=66, "MAG_Z"=68, "PRESSURE_I"=70, "PRESSURE_D"=72, "PRESSURE_TEMP"=74, "YAW_OFFSET"=76, "QUAT_OFFSET_W"=78, "QUAT_OFFSET_X"=80, "QUAT_OFFSET_Y"=82, "QUAT_OFFSET_Z"=84] ("Device Register (WHOAMI)")
            n259 = global read "Global Variables.vi" "NavX"() -> (w404:string)
            n260 = global read "Global Variables.vi" "NavX"() -> (w381:string)
            n261 = call "navX GetRefnum.vi"("refnum name"=w404) -> ("navX Device TypeDef"=w405:T6)  [unwired: 9 in, 1 out]
            n262 = call "navX GetRefnum.vi"("refnum name"=w381) -> ("navX Device TypeDef"=w380:T6)  [unwired: 9 in, 1 out]
            n263 = call "navX Read.vi"("Device Register (WHOAMI)"=w403, "navX Device TypeDef"=w405) -> ("navX Data"=w395:u8[])  [unwired: 7 in, 2 out]
            n264 = call "navX Read.vi"("Device Register (WHOAMI)"=w382, "navX Device TypeDef"=w380) -> ("navX Data"=w390:u8[])  [unwired: 7 in, 2 out]
            n265 = Index Array(array=w395, index #1=0 ("index"), index #2=1 ("index")) -> (element #1=w397:u8, element #2=w396:u8)
            n266 = Index Array(array=w390, index #1=0 ("index"), index #2=1 ("index")) -> (element #1=w388:u8, element #2=w389:u8)
            n267 = Join Numbers(hi=w396, lo=w397) -> ((hi.lo)=w400:u16)
            n268 = Join Numbers(hi=w389, lo=w388) -> ((hi.lo)=w385:u16)
            n269 = To Word Integer(number=w400) -> (16bit integer=w399:i16)
            n270 = To Word Integer(number=w385) -> (16bit integer=w386:i16)
            n271 = Divide(x=w399, y=i16 100) -> (x/y=w393:dbl)
            n272 = Divide(x=w386, y=i16 100) -> (x/y=w392:dbl)
            n273 = Absolute Value(x=w393) -> (abs(x)=w394:dbl)
            n274 = Absolute Value(x=w392) -> (abs(x)=w391:dbl)
          }
          frame Enabled {
            n275 = global read "Global Variables.vi" "NavX"() -> (w411:string)
            n276 = call "navX GetRefnum.vi"("refnum name"=w411) -> ("navX Device TypeDef"=w410:T6)  [unwired: 9 in, 1 out]
            n277 = call "GetYPRH.vi"("navX Device TypeDef"=w410) -> ("YPRH"=w412:T31)  [unwired: 8 in, 2 out]
            n278 = Unbundle By Name(w412) -> ("Yaw"=w407:dbl, "Pitch"=w409:dbl, "Roll"=w408:dbl, "Heading"=w406:dbl)
          }
        }
        n279 = Greater?(x=w378, y="Angle") -> (0:w376:bool)
        n280 = Greater?(x=w374, y="Angle") -> (0:w373:bool)
        n281 = Or(x=w376, y=w373) -> (x .or. y?=w375:bool)
        n282 = case shown="True" w375 {
          frame False {
          }
          frame True {
            n283 = local write "On Ramp"(TRUE ("On Ramp")) -> ()
          }
        }
        n284 = Bundle(cluster=cluster{"Pitch":dbl, "Roll":dbl} {"Pitch"=0.0, "Roll"=0.0}, "Pitch"=w353, "Roll"=w364) -> (w365:cluster{"Pitch":dbl, "Roll":dbl})
        n285 = Bundle(cluster=cluster{"Pitch":dbl, "Roll":dbl} {"Pitch"=0.0, "Roll"=0.0}, "Pitch"=w353, "Roll"=w356) -> (w361:cluster{"Pitch":dbl, "Roll":dbl})
        n286 = Bundle(cluster=cluster{"Pitch":dbl, "Roll":dbl} {"Pitch"=0.0, "Roll"=0.0}, "Pitch"=w353, "Roll"=w357) -> (w358:cluster{"Pitch":dbl, "Roll":dbl})
        n287 = Insert Into Array(array=w362, new element=w365) -> (w363:cluster{"Pitch":dbl, "Roll":dbl}[])  [unwired: 1 in]
        "Roll" <- w363
        n288 = Insert Into Array(array=w355, new element=w361) -> (w352:cluster{"Pitch":dbl, "Roll":dbl}[])  [unwired: 1 in]
        "Heading" <- w352
        n289 = Insert Into Array(array=w354, new element=w358) -> (w351:cluster{"Pitch":dbl, "Roll":dbl}[])  [unwired: 1 in]
        "Yaw" <- w351
        n290 = Bundle(cluster=cluster{"Pitch":dbl, "Roll":dbl} {"Pitch"=0.0, "Roll"=0.0}, "Pitch"=w353, "Roll"=w367) -> (w370:cluster{"Pitch":dbl, "Roll":dbl})
        n291 = Insert Into Array(array=w368, new element=w370) -> (w369:cluster{"Pitch":dbl, "Roll":dbl}[])  [unwired: 1 in]
        "Pitch" <- w369
        n292 = call "Wait2"("Count(mSec)"=u32 20) -> ()  [unwired: 1 out]
      }
    }
    frame Enabled {
    }
  }
  n293 = while {
    stop <- FALSE stop-if-true
    n294 = global read "Global Variables.vi" "Tachometer Dist New"() -> (w420:string)
    n295 = global read "Global Variables.vi" "Tachometer Dist"() -> (w424:string)
    n296 = global read "Global Variables.vi" "Tachometer BR"() -> (w440:string)
    n297 = global read "Global Variables.vi" "Tachometer FR"() -> (w428:string)
    n298 = global read "Global Variables.vi" "Tachometer FL"() -> (w439:string)
    n299 = global read "Global Variables.vi" "Tachometer BL"() -> (w452:string)
    n300 = Wait (ms)(milliseconds to wait=u32 5) -> ()  [unwired: 1 out]
    n301 = global read "Global Variables.vi" "Reset Tachs"() -> (w451:bool)
    n302 = call <vilib>:"WPI_CounterRefNum Registry Get.vi"("refnum name"=w424) -> ("error out"=w422:errorcluster, "CounterDevRef"=w426:T32)  [unwired: 9 in]
    n303 = call <vilib>:"WPI_CounterRefNum Registry Get.vi"("refnum name"=w428) -> ("error out"=w430:errorcluster, "CounterDevRef"=w429:T32)  [unwired: 9 in]
    n304 = call <vilib>:"WPI_CounterRefNum Registry Get.vi"("refnum name"=w440) -> ("error out"=w442:errorcluster, "CounterDevRef"=w441:T32)  [unwired: 9 in]
    n305 = call <vilib>:"WPI_CounterRefNum Registry Get.vi"("refnum name"=w439) -> ("error out"=w437:errorcluster, "CounterDevRef"=w438:T32)  [unwired: 9 in]
    n306 = call <vilib>:"WPI_CounterRefNum Registry Get.vi"("refnum name"=w420) -> ("error out"=w415:errorcluster, "CounterDevRef"=w418:T32)  [unwired: 9 in]
    n307 = call <vilib>:"WPI_CounterRefNum Registry Get.vi"("refnum name"=w452) -> ("error out"=w449:errorcluster, "CounterDevRef"=w450:T32)  [unwired: 9 in]
    n308 = case shown="True" w451 {
      tunnel: w450 -> [w464 w488]
      tunnel: w449 -> [w463 w487]
      tunnel: [w464 w486] -> w448
      tunnel: [w463 w485] -> w447
      tunnel: w441 -> [w461 w475]
      tunnel: w442 -> [w462 w484]
      tunnel: [w461 w474] -> w443
      tunnel: [w462 w473] -> w444
      tunnel: w438 -> [w460 w476]
      tunnel: w437 -> [w459 w483]
      tunnel: [w460 w477] -> w436
      tunnel: [w459 w478] -> w435
      tunnel: w429 -> [w457 w481]
      tunnel: w430 -> [w458 w482]
      tunnel: [w457 w480] -> w431
      tunnel: [w458 w479] -> w432
      tunnel: w426 -> [w456 w472]
      tunnel: [w456 w471] -> w425
      tunnel: w422 -> [w455 w470]
      tunnel: [w455 w469] -> w421
      tunnel: w418 -> [w454 w468]
      tunnel: [w454 w467] -> w417
      tunnel: [w453 w466] -> w416
      tunnel: w415 -> [w453 w465]
      frame False {
      }
      frame True {
        n309 = call <vilib>:"WPI_CounterReset.vi"("error in (no error)"=w483, "CounterDevRef in"=w476) -> ("error out"=w478:errorcluster, "CounterDevRef out"=w477:T32)  [unwired: 8 in]
        n310 = call <vilib>:"WPI_CounterReset.vi"("error in (no error)"=w482, "CounterDevRef in"=w481) -> ("error out"=w479:errorcluster, "CounterDevRef out"=w480:T32)  [unwired: 8 in]
        n311 = call <vilib>:"WPI_CounterReset.vi"("error in (no error)"=w484, "CounterDevRef in"=w475) -> ("error out"=w473:errorcluster, "CounterDevRef out"=w474:T32)  [unwired: 8 in]
        n312 = call <vilib>:"WPI_CounterReset.vi"("error in (no error)"=w470, "CounterDevRef in"=w472) -> ("error out"=w469:errorcluster, "CounterDevRef out"=w471:T32)  [unwired: 8 in]
        n313 = call <vilib>:"WPI_CounterReset.vi"("error in (no error)"=w487, "CounterDevRef in"=w488) -> ("error out"=w485:errorcluster, "CounterDevRef out"=w486:T32)  [unwired: 8 in]
        n314 = call <vilib>:"WPI_CounterReset.vi"("error in (no error)"=w465, "CounterDevRef in"=w468) -> ("error out"=w466:errorcluster, "CounterDevRef out"=w467:T32)  [unwired: 8 in]
      }
    }
    n315 = call <vilib>:"WPI_CounterGet.vi"("error in (no error)"=w432, "CounterDevRef in"=w431) -> ("Value"=w433:i32)  [unwired: 4 in, 5 out]
    n316 = call <vilib>:"WPI_CounterGet.vi"("error in (no error)"=w421, "CounterDevRef in"=w425) -> ("Value"=w423:i32)  [unwired: 4 in, 5 out]
    n317 = call <vilib>:"WPI_CounterGet.vi"("error in (no error)"=w416, "CounterDevRef in"=w417) -> ("Value"=w419:i32)  [unwired: 4 in, 5 out]
    n318 = call <vilib>:"WPI_CounterGet.vi"("error in (no error)"=w444, "CounterDevRef in"=w443) -> ("Value"=w445:i32)  [unwired: 4 in, 5 out]
    n319 = call <vilib>:"WPI_CounterGet.vi"("error in (no error)"=w435, "CounterDevRef in"=w436) -> ("Value"=w434:i32)  [unwired: 4 in, 5 out]
    n320 = call <vilib>:"WPI_CounterGet.vi"("error in (no error)"=w447, "CounterDevRef in"=w448) -> ("Value"=w446:i32)  [unwired: 4 in, 5 out]
    n321 = global write "Global Variables.vi" "Tach Dist"(w423) -> ()
    n322 = global write "Global Variables.vi" "Tach Dist New"(w419) -> ()
    n323 = global write "Global Variables.vi" "Tach BR"(w445) -> ()
    n324 = global write "Global Variables.vi" "Tach FR"(w433) -> ()
    n325 = global write "Global Variables.vi" "Tach FL"(w434) -> ()
    n326 = global write "Global Variables.vi" "Tach BL"(w446) -> ()
  }
